vi "Notification.vi"(8 "error in (no error)":errorcluster, 11 "NotificationBarString":string="Test") -> (0 "error out":errorcluster)   [LabVIEW 2012]
uses:
  <vilib>/Utility/miscctls.llb/LVRectTypeDef.ctl
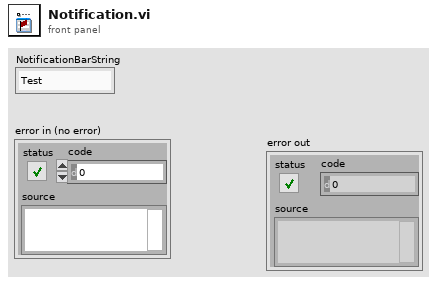
[diagram p1: front panel]
types:
  T1 = enum32{"Invalid", "Standard", "Closed", "Hidden", "Minimized", "Maximized"}
  T2 = typedef "LVRectTypeDef.ctl" = cluster{"Left":i16, "Top":i16, "Right":i16, "Bottom":i16}
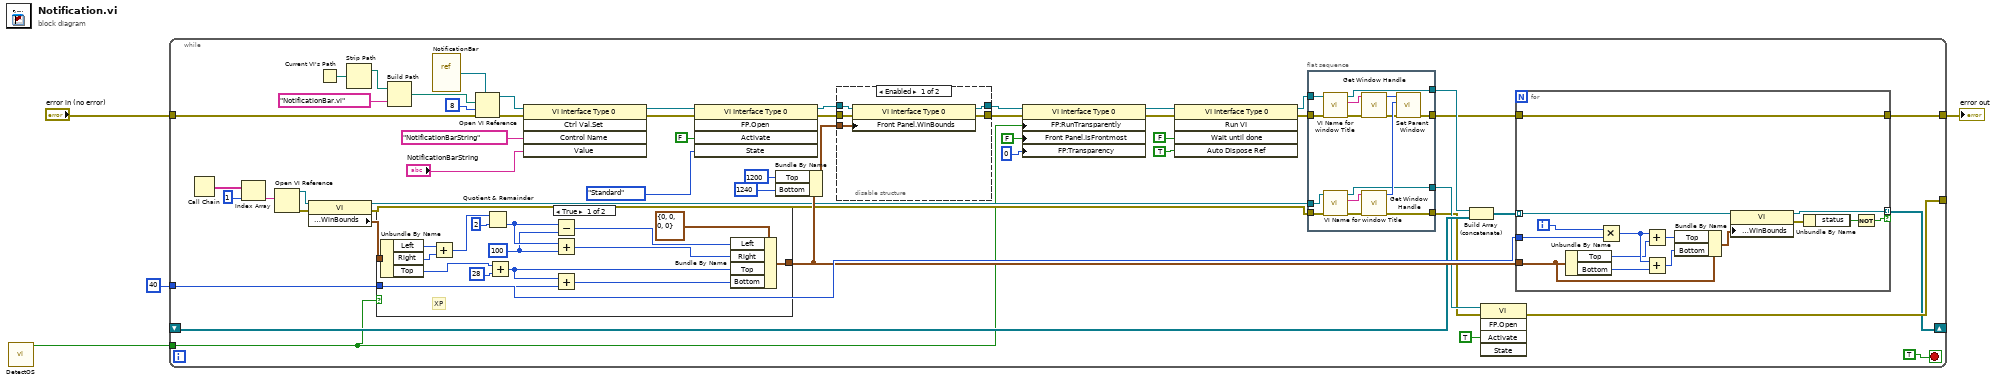
[diagram p0: block diagram]
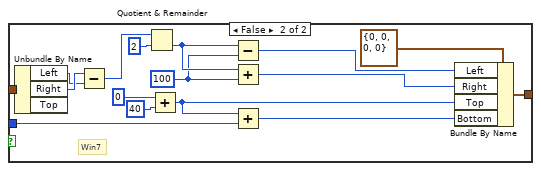
[diagram p2: hidden frame]
diagram:
  n1 = call "DetectOS.vi"() -> ("XP?"=w1:bool)  [unwired: 11 in]
  n2 = while {
    shift-right: [w14] -> _
    shift-left: _ -> [w16]
    tunnel: "error in (no error)" -> [w46]
    tunnel: [w19] -> w3
    tunnel: i16 40 ("x") -> [w30]
    tunnel: [w18] -> _
    tunnel: w1 -> [w5]
    stop <- TRUE stop-if-true
    n3 = Call Chain() -> (call chain=w56:string[])
    n4 = Index Array(array=w56, index=1) -> (element=w54:string)
    n5 = Open VI Reference(vi path=w54) -> (vi reference=w29:refnum<vi>, error out=w22:errorcluster)  [unwired: 5 in]
    n6 = property class="VI"(reference=w29, error in=w22) -> (reference out=w13:refnum<vi>, error out=w11:errorcluster, "Front Panel.WinBounds"=w35:T2)
    n7 = Current VI's Path() -> (path=w45:path)
    n8 = Strip Path(path=w45) -> (stripped path=w44:path)  [unwired: 1 out]
    n9 = case shown="True" w5 {
      tunnel: w35 -> [w72 w88]
      tunnel: w30 -> [w64 w80]
      tunnel: [w58 w74] -> w26
      frame True {
        w70 = i16 100 ("y")
        # "XP"
        n10 = Unbundle By Name(w72) -> ("Left"=w65:i16, "Right"=w66:i16, "Top"=w57:i16)
        n11 = Add(x=w65, y=w66) -> (x+y=w67:i16)
        n12 = Quotient & Remainder(x=w67, y=i16 2) -> (floor(x/y)=w71:i16)  [unwired: 1 out]
        n13 = Add(x=w57, y=i16 28) -> (x+y=w60:i16)
        n14 = Subtract(x=w71, y=w70) -> (x-y=w62:i16)
        n15 = Add(x=w71, y=w70) -> (x+y=w61:i16)
        n16 = Add(x=w60, y=w64) -> (x+y=w59:i16)
        n17 = Bundle By Name(cluster=T2 {"Left"=0, "Top"=0, "Right"=0, "Bottom"=0} ("Front Panel Window:Window Bounds"), "Left"=w62, "Right"=w61, "Top"=w60, "Bottom"=w59) -> (w58:T2)
      }
      frame False {
        w86 = i16 100 ("y")
        # "Win7"
        n18 = Unbundle By Name(w88) -> ("Left"=w81:i16, "Right"=w82:i16)  [unwired: 1 out]
        n19 = Subtract(x=w82, y=w81) -> (x-y=w83:i16)
        n20 = Quotient & Remainder(x=w83, y=i16 2) -> (floor(x/y)=w87:i16)  [unwired: 1 out]
        n21 = Add(x=i16 0, y=i16 40) -> (x+y=w76:i16)
        n22 = Subtract(x=w87, y=w86) -> (x-y=w78:i16)
        n23 = Add(x=w87, y=w86) -> (x+y=w77:i16)
        n24 = Add(x=w76, y=w80) -> (x+y=w75:i16)
        n25 = Bundle By Name(cluster=T2 {"Left"=0, "Top"=0, "Right"=0, "Bottom"=0} ("Front Panel Window:Window Bounds"), "Left"=w78, "Right"=w77, "Top"=w76, "Bottom"=w75) -> (w74:T2)
      }
    }
    n26 = Build Path(base path=w44, name or relative path="NotificationBar.vi") -> (appended path=w43:path)
    n27 = vi-ref "NotificationBar.vi"() -> (w53:refnum<vi>)
    n28 = Open VI Reference(type specifier VI Refnum (for type only)=w53, vi path=w43, options=8, error in (no error)=w46) -> (vi reference=w32:refnum<vi>, error out=w31:errorcluster)  [unwired: 2 in]
    n29 = invoke class="VI Interface Type 0" method="Ctrl Val.Set"(reference=w32, error in=w31, "Control Name"="NotificationBarString", "Value"="NotificationBarString") -> (reference out=w24:refnum<vi>, error out=w21:errorcluster)  [unwired: 1 in, 3 out]
    n30 = invoke class="VI Interface Type 0" method="FP.Open"(reference=w24, error in=w21, "Activate"=FALSE ("Activate?"), "State"=T1."Standard") -> (reference out=w38:refnum<vi>, error out=w40:errorcluster)  [unwired: 1 in, 3 out]
    n31 = Bundle By Name(cluster=w26, "Top"=i16 1200, "Bottom"=i16 1240) -> (w9:T2)
    n32 = disable-structure shown="Enabled" {
      disable-tunnel: w40 -> [w93 _]
      disable-tunnel: w38 -> [w92 w94]
      disable-tunnel: [w91 _] -> w36
      disable-tunnel: [w90 w94] -> w34
      disable-tunnel: w9 -> [w89 _]
      frame Enabled {
        n33 = property class="VI Interface Type 0"(reference=w92, error in=w93, "Front Panel.WinBounds"=w89) -> (reference out=w90:refnum<vi>, error out=w91:errorcluster)
      }
      frame Disabled {
      }
    }
    n34 = property class="VI Interface Type 0"(reference=w34, error in=w36, "FP:RunTransparently"=w5, "Front Panel.IsFrontmost"=FALSE ("Front Panel Window:Is Frontmost"), "FP:Transparency"=u8 0 ("Front Panel Window:Transparency")) -> (reference out=w23:refnum<vi>, error out=w17:errorcluster)
    n35 = invoke class="VI Interface Type 0" method="Run VI"(reference=w23, error in=w17, "Wait until done"=FALSE ("Wait Until Done"), "Auto Dispose Ref"=TRUE ("Auto Dispose Reference")) -> (reference out=w28:refnum<vi>, error out=w20:errorcluster)  [unwired: 1 in, 3 out]
    n36 = flat-sequence {
      tunnel: w13 -> [w104]
      tunnel: w28 -> [w103]
      tunnel: [w102] -> w27
      tunnel: [w101] -> w25
      tunnel: w20 -> [w100]
      tunnel: [w98] -> w12
      tunnel: w11 -> [w97]
      tunnel: [w95] -> w10
      frame #0 {
        n37 = call "VI Name for window Title.vi"("error in"=w100, "vi reference"=w103) -> ("error out"=w105:errorcluster, "Vi tiltle"=w108:string, "vi reference out (dup)"=w102:refnum<vi>)  [unwired: 7 out]
        n38 = call "VI Name for window Title.vi"("error in"=w97, "vi reference"=w104) -> ("error out"=w99:errorcluster, "Vi tiltle"=w109:string, "vi reference out (dup)"=w98:refnum<vi>)  [unwired: 7 out]
        n39 = call "Get Window Handle.vi"("error in (no error)"=w105, "window name (\"\")"=w108) -> ("error out"=w96:errorcluster, "hWnd"=w106:u32)  [unwired: 1 in, 3 out]
        n40 = call "Get Window Handle.vi"("error in (no error)"=w99, "window name (\"\")"=w109) -> ("error out"=w95:errorcluster, "hWnd"=w107:u32)  [unwired: 1 in, 3 out]
        n41 = call "Set Parent Window.vi"("error in (no error)"=w96, "new parent"=w107, "child"=w106) -> ("error out"=w101:errorcluster)  [unwired: 1 in, 7 out]
      }
    }
    n42 = Build Array (concatenate)(w27, w16) -> (w15:refnum<vi>[])
    n43 = invoke class="VI" method="FP.Open"(reference=w12, error in=w10, "Activate"=TRUE ("Activate?")) -> (error out=w18:errorcluster)  [unwired: 2 in, 4 out]
    n44 = for {
      tunnel: w15 -> [w115] mode=indexing
      tunnel: [w121] -> w14 mode=indexing if=w118
      tunnel: w30 -> [w117]
      tunnel: w26 -> [w114]
      tunnel: w25 -> [w111]
      tunnel: [w111] -> w19
      i -> [w110]
      n45 = Unbundle By Name(w114) -> ("Top"=w113:i16, "Bottom"=w112:i16)
      n46 = Multiply(x=w110, y=w117) -> (x*y=w116:i32)
      n47 = Add(x=w116, y=w113) -> (x+y=w123:i32)
      n48 = Add(x=w116, y=w112) -> (x+y=w122:i32)
      n49 = Bundle By Name(cluster=w114, "Top"=w123, "Bottom"=w122) -> (w124:T2)
      n50 = property class="VI"(reference=w115, "Front Panel.WinBounds"=w124) -> (reference out=w121:refnum<vi>, error out=w120:errorcluster)  [unwired: 1 in]
      n51 = Unbundle By Name(w120) -> ("status"=w119:bool)
      n52 = Not(x=w119) -> (.not. x?=w118:bool)
    }
  }
  "error out" <- w3
